vi "TEST - Dist Build App from LLB (proxy).vi"(8 "error in (no error)":errorcluster) -> (0 "error out":errorcluster, 2 "pass":bool)   [LabVIEW 2020]
uses:
  <userlib>/_OpenG.lib/file/file.llb/Convert File Extension (Path)__ogtk.vi
  <userlib>/_OpenG.lib/error/error.llb/openg_error.lvlib
  <userlib>/_OpenG.lib/file/file.llb/openg_file.lvlib
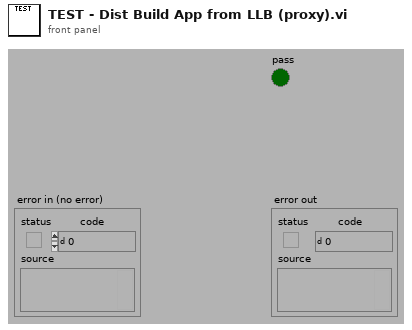
[diagram p1: front panel]
types:
  T1 = cluster{"destination executable":path, "source llb":path, "source shell":path, "custom icon":path}
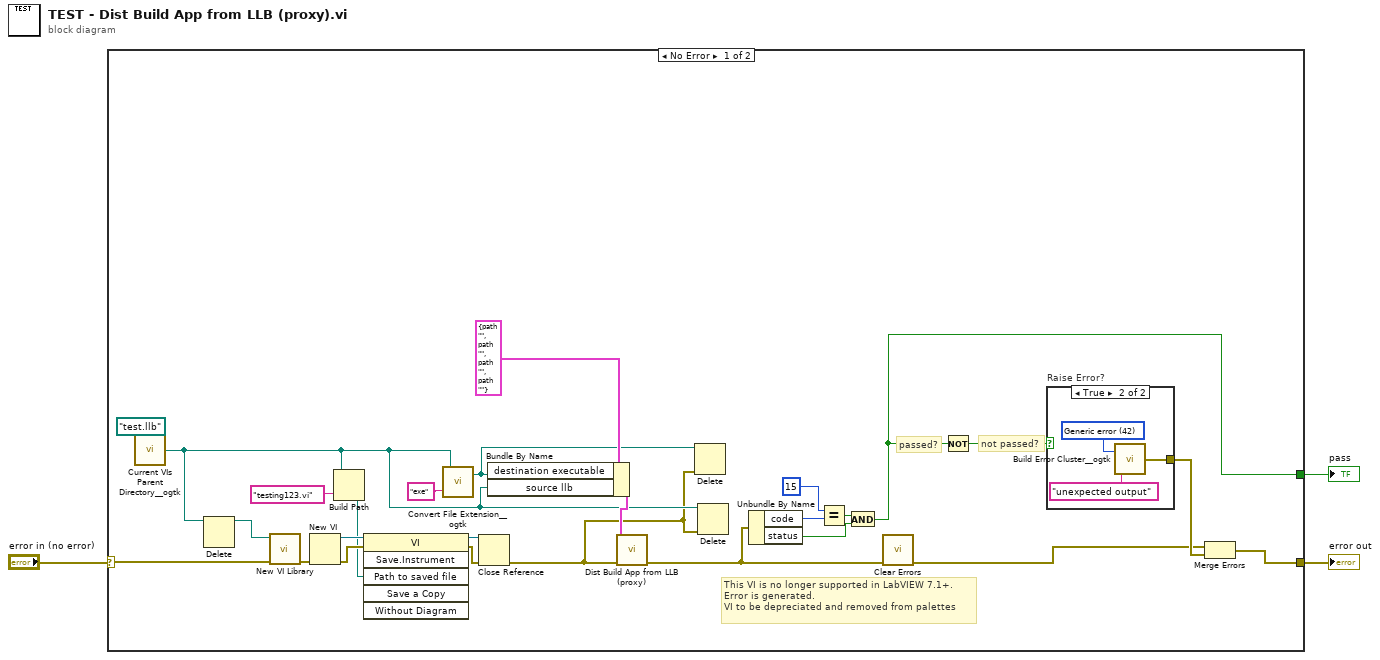
[diagram p0: block diagram]
diagram:
  n1 = case shown="No Error" "error in (no error)" {
    selector: "error in (no error)" -> [w18 w33]
    tunnel: [w7 _] -> w3
    tunnel: [w29 w33] -> w1
    frame No Error {
      # "This VI is no longer supported in LabVIEW 7.1+.\nError is generated.\nVI to be depreciated and removed from palettes"
      # "not passed?"
      # "passed?"
      n2 = call <userlib>:"Current VIs Parent Directory__ogtk.vi"("Relative path (.)"=path "test.llb") -> ("Parent Directory (+ Relative)"=w12:path)  [unwired: 4 in]
      n3 = Delete(path (use dialog)=w12) -> (deleted path=w14:path)  [unwired: 4 in, 2 out]
      n4 = call <vilib>:"New VI Library.vi"("error in (no error)"=w18, "VI library path in"=w14) -> ("error out"=w25:errorcluster)  [unwired: 8 in, 1 out]
      n5 = New VI(8:w25) -> (0:w24:errorcluster, 3:w23:refnum<vi>)  [unwired: 6 in]
      n6 = Build Path(base path=w12, name or relative path="testing123.vi") -> (appended path=w21:path)
      n7 = invoke class="VI" method="Save.Instrument"(reference=w23, error in=w24, "Path to saved file"=w21) -> (reference out=w20:refnum<vi>, error out=w19:errorcluster)  [unwired: 3 in, 4 out]
      n8 = call-poly <userlib>:"Convert File Extension__ogtk.vi"("new ending (none)"="exe", "file name"=w12) -> ("new filename"=w13:path)  [unwired: 1 out]
      n9 = Close Reference(reference=w20, error in (no error)=w19) -> (error out=w4:errorcluster)
      n10 = Bundle By Name(cluster=T1 {"destination executable"=path "", "source llb"=path "", "source shell"=path "", "custom icon"=path ""} ("paths"), "destination executable"=w13, "source llb"=w12) -> (w15:T1)
      n11 = call "Dist Build App from LLB (proxy).vi"("error in"=w4, "paths"=w15) -> ("error out"=w6:errorcluster)  [unwired: 9 in]
      n12 = Delete(path (use dialog)=w13, error in=w4) -> ()  [unwired: 3 in, 3 out]
      n13 = Delete(path (use dialog)=w12, error in=w4) -> ()  [unwired: 3 in, 3 out]
      n14 = Unbundle By Name(w6) -> ("code"=w11:i32, "status"=w8:bool)
      n15 = Equal?(x=15, y=w11) -> (x = y?=w9:bool)
      n16 = And(x=w9, y=w8) -> (x .and. y?=w7:bool)
      n17 = call <vilib>:"Clear Errors.vi"("error in (no error)"=w6) -> ("error out"=w5:errorcluster)  [unwired: 5 in, 1 out]
      n18 = Not(x=w7) -> (.not. x?=w27:bool)
      n19 = case "Raise Error?" shown="True" w27 {
        tunnel: [_ w30] -> w28
        frame False {
        }
        frame True {
          w31 = 42 items=["No error", "Argument error", "Memory is full", "Out of zone", "End of file", "File already open", "Generic file I/O error", "File not found", "File permission error", "Disk is full", "Duplicate path", "Too many files open", "System feature not enabled", "Resource file not found", "Cannot add resource", "Resource not found", "Image not found", "Image memory error", "Pen does not exist", "Config type invalid", "Config token not found", "Config parse error", "Config memory error", "Bad external code format", "Bad external code offset", "External code not present", "Null window", "Destroy window error", "Null menu", "Print aborted", "Bad print record", "Print driver error", "Windows error during printing", "Memory error during printing", "Print dialog error", "Generic print error", "Invalid device refnum", "Device not found", "Device parameter error", "Device unit error", "Cannot open device", "Device call aborted", "Generic error", "Cancelled by user", "Object ID too low", "Object ID too high", "Object not in heap", "Unknown heap", "Unknown object (invalid DefProc)", "Unknown object (DefProc not in table)", "Message out of range", "Invalid (null) method", "Unknown message", "Manager call not supported", "Bad address", "Network operation in progress", "Network operation timed out", "Connection is busy", "Network attribute not supported", "Network error", "Address in use", "System out of memory", "Connection aborted", "Connection refused", "Not connected", "Already connected", "Connection closed", "Initialization error (interapplication manager)", "Bad occurrence", "Wait on unbound occurrence handler", "Occurrence queue overflow", "Datalog type conflict", "Unused", "Unrecognized type (interapplication manager)", "Memory corrupt", "Failed to make temporary DLL", "Old CIN version", "Drag socket not found", "Failed to load drop-object", "Failed to register OLE object", "Failed to release OLE object", "Format specifier type mismatch", "Unknown format specifier", "Too few format specifiers", "Too many format specifiers", "Scan failed", "Newer CIN version", "Error converting to variant", "Runtime menu error", "Password tampered", "Variant attribute not found", "Incompatible variant data type", "Event data is not available", "Event Store is not present", "Occurrence is not found", "Event Queue is not created", "Event info is not available", "Refnum passed is NULL", "Error retrieving Class GUID", "Error retrieving CoClass GUID", "Error retrieving TypeLib GUID.", "Bad built application magic bytes.", "Specific driver is different from the specific driver associated with the Logical Name.", "There is no session opened to the class driver.", "Max Error", "MAX - Error with config objects", "MAX - Error loading configuration", "MAX - Group not supported"]
          n20 = call <userlib>:"Build Error Cluster__ogtk.vi"("String to Prepend to source (\"\")"="unexpected output" ("String to Prepend to source (\"\")"), "code"=w31) -> ("error out"=w30:errorcluster)
        }
      }
      n21 = Merge Errors(w5, w28) -> (w29:errorcluster)
    }
    frame Error {
    }
  }
  "pass" <- w3
  "error out" <- w1
